vi "InitiateMIPI_RFFE.vi"(8 "error in (no error)":errorcluster, 11 "Configuratation In":T3={"Samples to Allocate"=10000, "Oversample Factor"=1, "Clock Channel"=enum."0", "Data Channel"=enum."1"} {"Oversample Factor" min=1 max=254; "Samples to Allocate" min=1}) -> (0 "error out":errorcluster, 1 "Number of Samples Out":i32, 2 "Data Array":u8[][](array[numeric]), 3 "RFFE_Data":T1 {"Toggle (high to low)" items=["0", "1", "Z", "L", "H", "X", "T", "V"]; "X Array" items=["0", "1", "Z", "L", "H", "X", "T", "V"]; "Z Array" items=["0", "1", "Z", "L", "H", "X", "T", "V"]; "L Array" items=["0", "1", "Z", "L", "H", "X", "T", "V"]; "H Array" items=["0", "1", "Z", "L", "H", "X", "T", "V"]; "One Array" items=["0", "1", "Z", "L", "H", "X", "T", "V"]; "Zero Array" items=["0", "1", "Z", "L", "H", "X", "T", "V"]})   [LabVIEW 2013]
doc: "Peeallocates arrays and initializes values."
uses:
  Ctrls/Configuration.ctl
  Ctrls/ClockDataChannels.ctl
  Ctrls/RFFE_Data.ctl
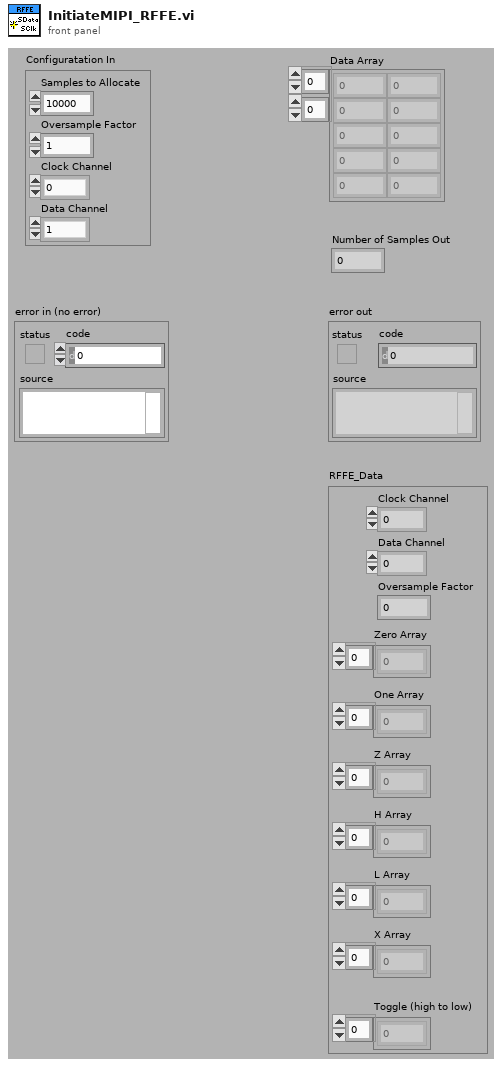
[diagram p1: front panel]
types:
  T1 = typedef "RFFE_Data.ctl" = cluster{"Clock Channel":T2, "Data Channel":T2, "Oversample Factor":u8, "Zero Array":u8[], "One Array":u8[], "Z Array ":u8[], "H Array":u8[], "L Array":u8[], "X Array":u8[], "Toggle (high to low)":u8[]}
  T2 = typedef "ClockDataChannels.ctl" = enum16{"0", "1"}
  T3 = typedef "Configuration.ctl" = cluster{"Samples to Allocate":i32, "Oversample Factor":u8, "Clock Channel":T2, "Data Channel":T2}
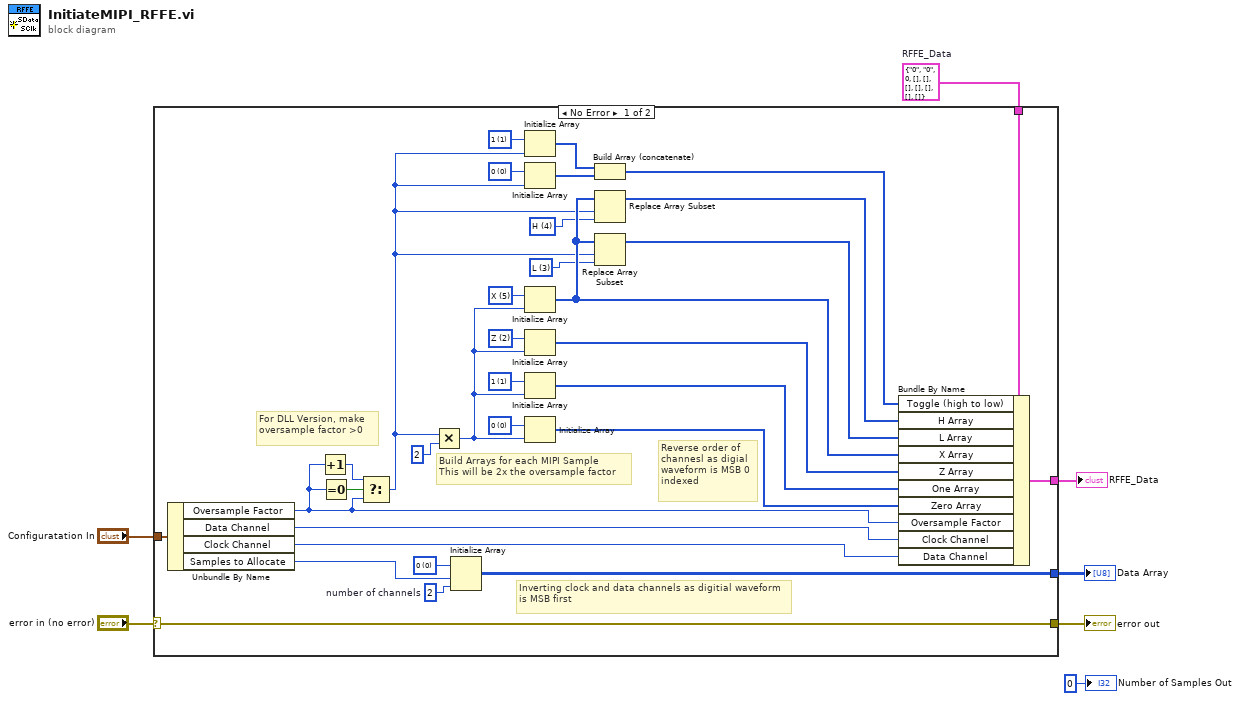
[diagram p0: block diagram]
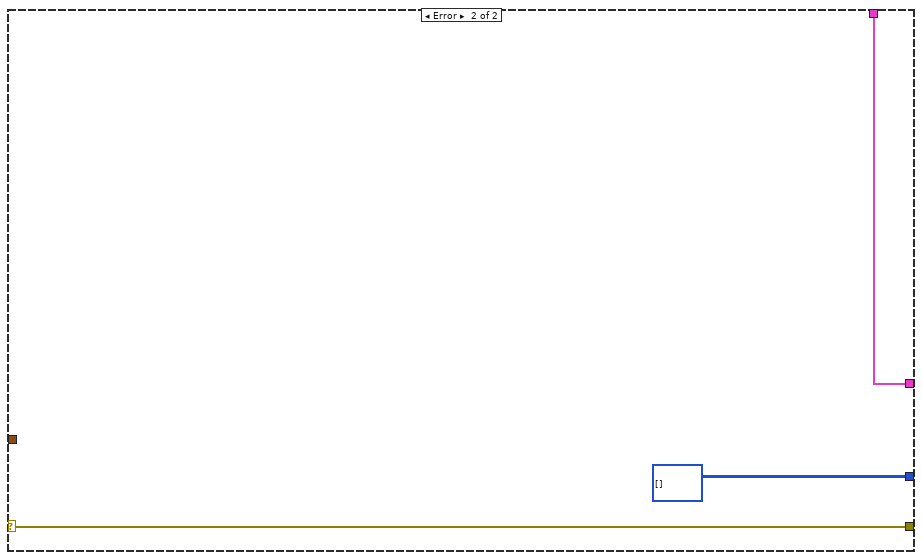
[diagram p2: hidden frame]
diagram:
  w2 = T1 {"Clock Channel"=enum."0", "Data Channel"=enum."0", "Oversample Factor"=0, "Zero Array"=[], "One Array"=[], "Z Array "=[], "H Array"=[], "L Array"=[], "X Array"=[], "Toggle (high to low)"=[]}  # RFFE_Data
  n1 = case shown="No Error" "error in (no error)" {
    selector: "error in (no error)" -> [w34 w43]
    tunnel: [w34 w43] -> w5
    tunnel: [w38 u8[][] []] -> w6
    tunnel: "Configuratation In" -> [w24 _]
    tunnel: [w37 w41] -> w3
    tunnel: w2 -> [w36 w41]
    frame No Error {
      w17 = u8 0 items=["0", "1", "Z", "L", "H", "X", "T", "V"] ("digital values ring")
      w18 = u8 1 items=["0", "1", "Z", "L", "H", "X", "T", "V"] ("digital values ring")
      w21 = u8 4 items=["0", "1", "Z", "L", "H", "X", "T", "V"] ("digital values ring")
      w22 = u8 3 items=["0", "1", "Z", "L", "H", "X", "T", "V"] ("digital values ring")
      w25 = u8 5 items=["0", "1", "Z", "L", "H", "X", "T", "V"] ("digital values ring")
      w26 = u8 2 items=["0", "1", "Z", "L", "H", "X", "T", "V"] ("digital values ring")
      w30 = u8 1 items=["0", "1", "Z", "L", "H", "X", "T", "V"] ("digital values ring")
      w32 = u8 0 items=["0", "1", "Z", "L", "H", "X", "T", "V"] ("digital values ring")
      w39 = 2  # number of channels
      w40 = u8 0 items=["0", "1", "Z", "L", "H", "X", "T", "V"] ("digital values ring")
      # "Build Arrays for each MIPI Sample\nThis will be 2x the oversample factor"
      # "For DLL Version, make oversample factor >0"
      # "Inverting clock and data channels as digitial waveform is MSB first"
      # "Reverse order of channesl as digial waveform is MSB 0 indexed"
      n2 = Unbundle By Name(w24) -> ("Oversample Factor"=w10:u8, "Data Channel"=w11:T2, "Clock Channel"=w15:T2, "Samples to Allocate"=w35:i32)
      n3 = Increment(x=w10) -> (x+1=w13:u8)
      n4 = Equal To 0?(x=w10) -> (x = 0?=w14:bool)
      n5 = Select(t=w13, s=w14, f=w10) -> (s? t:f=w12:u8)
      n6 = Multiply(x=w12, y=u8 2 ("x")) -> (x*y=w27:u8)
      n7 = Initialize Array(w40, w35, w39) -> (w38:u8[][])
      n8 = Initialize Array(w18, w12) -> (w9:u8[])
      n9 = Initialize Array(w17, w12) -> (w8:u8[])
      n10 = Initialize Array(w25, w27) -> (w23:u8[])
      n11 = Initialize Array(w26, w27) -> (w28:u8[])
      n12 = Initialize Array(w30, w27) -> (w29:u8[])
      n13 = Initialize Array(w32, w27) -> (w31:u8[])
      n14 = Build Array (concatenate)(w9, w8) -> (w16:u8[])
      n15 = Replace Array Subset(array=w23, new element=w21, index=w12) -> (w20:u8[])
      n16 = Replace Array Subset(array=w23, new element=w22, index=w12) -> (w19:u8[])
      n17 = Bundle By Name(cluster=w36, "Toggle (high to low)"=w16, "H Array"=w20, "L Array"=w19, "X Array"=w23, "Z Array"=w28, "One Array"=w29, "Zero Array"=w31, "Oversample Factor"=w10, "Clock Channel"=w11, "Data Channel"=w15) -> (w37:T1)
    }
    frame Error {
    }
  }
  "error out" <- w5
  "Data Array" <- w6
  "RFFE_Data" <- w3
  "Number of Samples Out" <- 0 ("Number of Samples Out")
